vi "LINX - Digital Write Square Wave.vi"() -> ()   [LabVIEW 2020]
doc: "This example demonstrates how to genrate a square wave using a LINX device."
uses:
  vi.lib/MakerHub/LINX/Public/Utilities/Open Serial.vi
  vi.lib/MakerHub/LINX/LMH-LINX.lvlib
panel:
  in  "Duration (ms)":u32
  in  "Frequency (Hz)":u32
  in  "DO Channel":u8=13
  in  "Stop Button":bool
  in  "Serial Port":refnum<visa-resource-name>
  # "Digital Write Square Wave Example\n\nThis example demonstrates how to generate a square wave with a user specified frequency.\n\nThe generated square wave will always have a 50% duty cylce.  The waveform will be \ngenerated for the specified duration (in ms) or until The Digital Write Square wave VI \nis called again.  A Duration of 0 stops the square wave output.\n\nInstructions\n1. Select the COM Port associated with the LINX Device.\n2. Select a supported Channel to generate a square wave on.\n3. Click the Run Arrow.\n4. Adjust the Frequency and Duration to control the square wave output."
  # "LINX Device Settings"
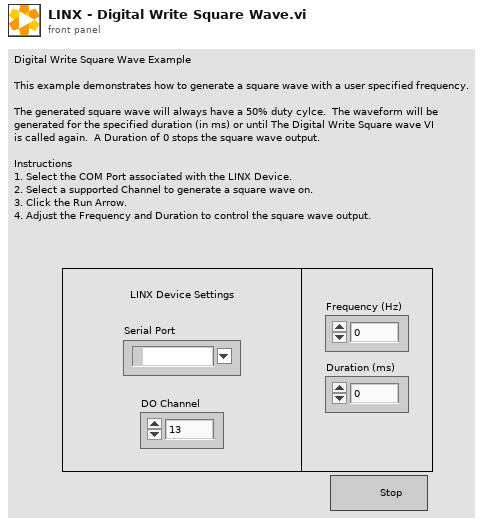
[diagram p1: front panel]
types:
  T1 = typedef "LMH-LINX.lvlib/LINX Ref.ctl" = cluster{"IO":T2, "Interface":T3, "LINX Device Config":T4}
  T2 = typedef "LMH-LINX.lvlib/Platform.ctl" = enum16{"Remote", "Local"}
  T3 = typedef "LMH-LINX.lvlib/Interface.ctl" = enum16{"Serial", "TCP"}
  T4 = typedef "Device.lvlib/LINX Device Config.ctl" = cluster{"Interface":T3, "COM Port":refnum<visa-resource-name>, "TCP Configuration":T5, "Device Family":u8, "Device ID":u8, "Device Name":string, "TCP Ref":refnum<k5>, "Channels":T6}
  T5 = typedef "Device.lvlib/TCP Config.ctl" = cluster{"IP Address":string, "Port":u16}
  T6 = typedef "LMH-LINX.lvlib/Channels.ctl" = cluster{"DI":u8[], "DO":u8[], "AI":u8[], "AO":u8[], "PWM":u8[], "QE":u8[], "UART":u8[], "I2C 2":u8[], "SPI":u8[], "CAN":u8[], "Servo":u8[], "AI Ref (V)":dbl, "AI Resolution (Bits)":u8, "AO Ref (V)":dbl, "AO Resolution (Bits)":u8}
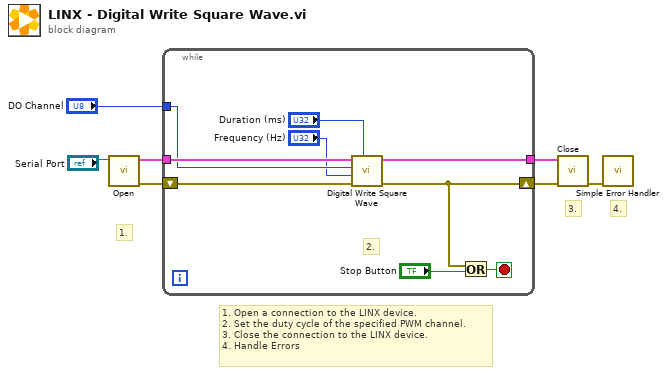
[diagram p0: block diagram]
diagram:
  # "1. Open a connection to the LINX device.\n2. Set the duty cycle of the specified PWM channel.\n3. Close the connection to the LINX device.\n4. Handle Errors"
  # "4."
  # "3."
  # "1."
  n1 = call-poly "Open.vi"("Serial Port"="Serial Port") -> ("Error Out"=w6:errorcluster, "LINX Resource"=w7:T1)  [unwired: 8 in, 1 out]
  n2 = while {
    tunnel: w7 -> [w13]
    tunnel: [w14] -> w5
    shift-right: [w12] -> w4
    shift-left: w6 -> [w11]
    tunnel: "DO Channel" -> [w10]
    stop <- w16 stop-if-true
    # "2."
    n3 = call "Digital Write Square Wave.vi"("Duration (ms)"="Duration (ms)", "Error In"=w11, "Frequency (Hz)"="Frequency (Hz)", "Channel"=w10, "LINX Resource"=w13) -> ("Error Out"=w12:errorcluster, "LINX Resource"=w14:T1)  [unwired: 5 in]
    n4 = Or(x=w12, y="Stop Button") -> (x .or. y?=w16:bool)
  }
  n5 = call "Close.vi"("Error In"=w4, "LINX Resource"=w5) -> ("Error Out"=w2:errorcluster)  [unwired: 9 in]
  n6 = call <vilib>:"Simple Error Handler.vi"("error in (no error)"=w2) -> ()  [unwired: 4 in, 5 out]
